vi "CONVERTERU32.vi"(11 "data":u32[](array[numeric])) -> (3 "Boolean array":bool[](array[boolean]))   [LabVIEW 2020, in "Acquisition.lvlib"]
uses:
  Acquisition.lvlib
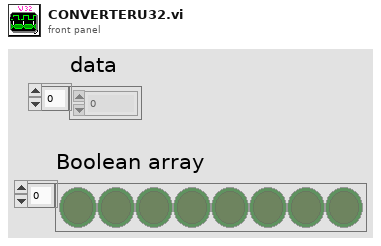
[diagram p1: front panel]
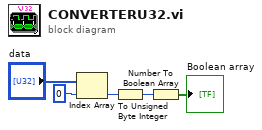
[diagram p0: block diagram]
diagram:
  n1 = Index Array(array="data", index=0) -> (element=w2:u32)
  n2 = To Unsigned Byte Integer(number=w2) -> (unsigned 8bit integer=w3:u8)
  n3 = Number To Boolean Array(number=w3) -> (Boolean array=→"Boolean array":bool[])
